vi "Get Array Elements.vi"(6 "Pass non-arrays":bool, 8 "error in (no error)":errorcluster, 10 "Offset":i32, 11 "JSON":string) -> (0 "error out":errorcluster, 1 "<JSON>":string[](array[string]) caption="<JSON>Elements", 2 "Offset past":i32 caption="Offset past Array")   [LabVIEW 2017, in "JSONtext.lvlib"]
doc: "If a JSON Array, returns all elements of the Array.\n\nIf the input JSON is not an Array, this function will return an error, unless \"Pass non-arrays\" is true, in which case the output will be a one-element array containing the input JSON."
uses:
  JSONtext.lvlib
  Parsing/Parsing State.ctl
  Parsing/Advance past String.vi
  Parsing/Advance past Number.vi
  Parsing/Advance past Array.vi
  Parsing/Advance past Object.vi
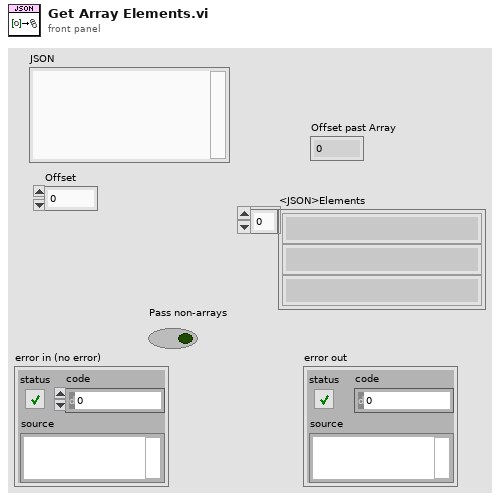
[diagram p1: front panel]
types:
  T1 = typedef "JSONtext.lvlib/Parsing State.ctl" = enum16{"Parser Error", "Object", "Array", "String", "Number/Other", "Leading Whitespace", "Object end", "Array end", "Value end"}
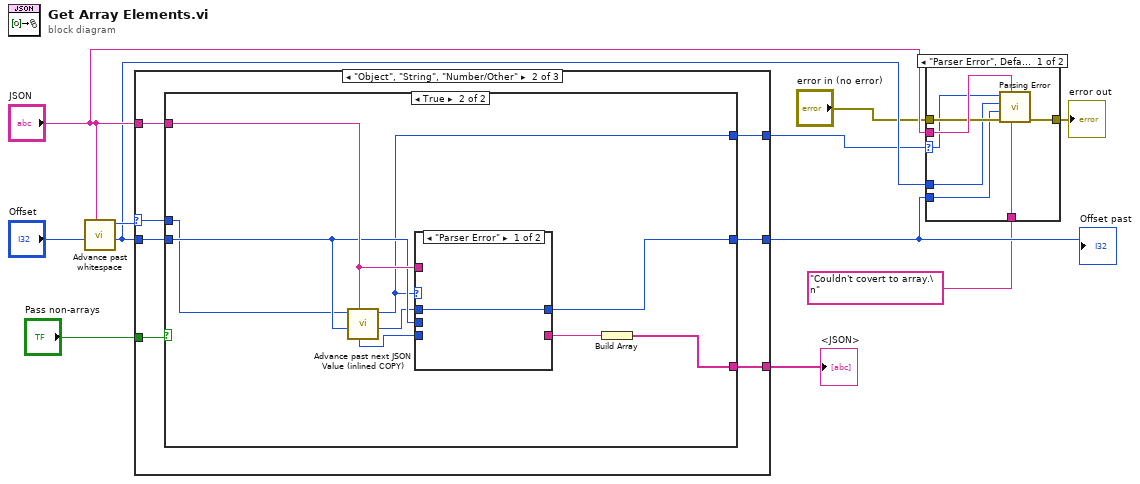
[diagram p0: block diagram]
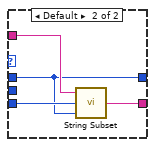
[diagram p5: hidden frame]
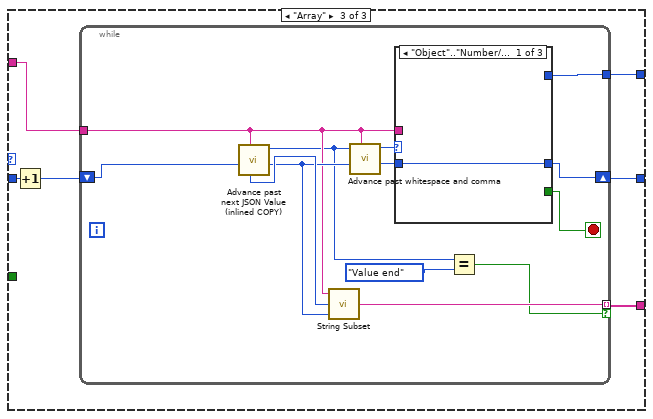
[diagram p6: hidden frame]
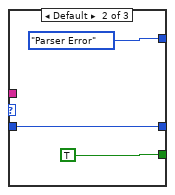
[diagram p7: hidden frame]
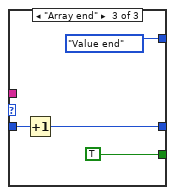
[diagram p8: hidden frame]
diagram:
  n1 = call "Advance past whitespace.vi"("JSON"="JSON", "Offset"="Offset") -> ("Offset of first non-whitespace"=w7:i32, "Parser State"=w9:T1)  [unwired: 8 in]
  n2 = case shown="\"Object\", \"String\", \"Number/Other\"" w9 {
    selector: w9 -> [w13 w14 _]
    tunnel: [w13 w16 w42] -> w3
    tunnel: [w12 w17 w41] -> w6
    tunnel: [_ w18 w39] -> w11
    tunnel: "JSON" -> [_ w20 w38]
    tunnel: w7 -> [w12 w19 w37]
    tunnel: "Pass non-arrays" -> [_ w15 _]
    frame "Parser Error", Default {
    }
    frame "Object", "String", "Number/Other" {
      n3 = case shown="True" w15 {
        tunnel: w20 -> [_ w31]
        tunnel: w19 -> [w21 w30]
        tunnel: [_ w26] -> w18
        tunnel: [w21 w25] -> w17
        tunnel: [w22 w24] -> w16
        tunnel: w14 -> [w22 w23]
        frame False {
        }
        frame True {
          n4 = call "Advance past next JSON Value (inlined COPY).vi"("JSON"=w31, "Offset"=w30, "State"=w23) -> ("Offset"=w29:i32, "State"=w24:T1, "Value start"=w28:i32)  [unwired: 4 in, 2 out]
          n5 = case shown="\"Parser Error\"" w24 {
            tunnel: w28 -> [_ w36]
            tunnel: w30 -> [_ _]
            tunnel: w29 -> [w32 w33]
            tunnel: [_ w35] -> w27
            tunnel: w31 -> [_ w34]
            tunnel: [w32 w33] -> w25
            frame "Parser Error" {
            }
            frame Default {
              n6 = call "String Subset.vi"("Offset past End"=w33, "Start offset"=w36, "JSON"=w34) -> ("substring"=w35:string)  [unwired: 2 in]
            }
          }
          n7 = Build Array(w27) -> (w26:string[])
        }
      }
    }
    frame "Array" {
      n8 = Increment(x=w37) -> (x+1=w40:i32)
      n9 = while {
        tunnel: w38 -> [w47]
        shift-right: [w52] -> w41
        shift-left: w40 -> [w53]
        tunnel: [w50] -> w42
        tunnel: [w44] -> w39 mode=indexing if=w43
        stop <- w51 stop-if-true
        n10 = call "Advance past next JSON Value (inlined COPY).vi"("JSON"=w47, "Offset"=w53) -> ("Offset"=w48:i32, "State"=w45:T1, "Value start"=w49:i32)  [unwired: 5 in, 2 out]
        n11 = call "String Subset.vi"("Offset past End"=w48, "Start offset"=w49, "JSON"=w47) -> ("substring"=w44:string)  [unwired: 2 in]
        n12 = call "Advance past whitespace and comma.vi"("JSON"=w47, "Offset"=w48, "State in"=w45) -> ("Offset past match"=w55:i32, "State"=w54:T1)  [unwired: 7 in]
        n13 = case shown="\"Object\"..\"Number/Other\"" w54 {
          tunnel: [_ TRUE TRUE] -> w51
          tunnel: [_ Parsing_State."Parser Error" Parsing_State."Value end"] -> w50
          tunnel: w55 -> [w56 w57 w61]
          tunnel: [w56 w57 w60] -> w52
          tunnel: w47 -> [_ _ _]
          frame "Object".."Number/Other" {
          }
          frame Default {
          }
          frame "Array end" {
            n14 = Increment(x=w61) -> (x+1=w60:i32)
          }
        }
        n15 = Equal?(x=w45, y=Parsing_State."Value end") -> (x = y?=w43:bool)
      }
    }
  }
  "Offset past" <- w6
  "<JSON>" <- w11
  n16 = case shown="\"Parser Error\", Default" w3 {
    selector: w3 -> [w65 _]
    tunnel: "JSON" -> [w70 _]
    tunnel: "error in (no error)" -> [w69 w71]
    tunnel: [w68 w71] -> w5
    tunnel: w7 -> [w67 _]
    tunnel: w6 -> [w66 _]
    tunnel: "Couldn't covert to array.\n" -> [w64 _]
    frame "Parser Error", Default {
      n17 = call "Parsing Error.vi"("initial string"=w64, "JSON"=w70, "error in (no error)"=w69, "Offset past match"=w66, "Value start"=w67, "State"=w65) -> ("error out"=w68:errorcluster)  [unwired: 5 in]
    }
    frame "Value end" {
    }
  }
  "error out" <- w5
